vi "Escape.vi"(11 "text":string) -> (3 "escaped text":string)   [LabVIEW 2021, in "HttpServer.lvlib"]
uses:
  HttpServer.lvlib
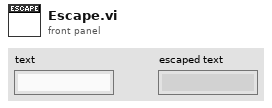
[diagram p1: front panel]
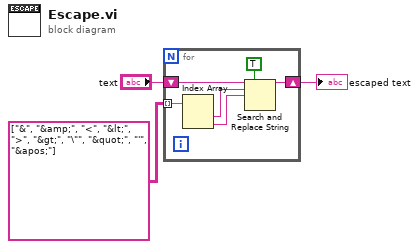
[diagram p0: block diagram]
diagram:
  n1 = for {
    tunnel: string[][] [["&", "&amp;"], ["<", "&lt;"], [">", "&gt;"], ["\"", "&quot;"], ["'", "&apos;"]] -> [w7] mode=indexing
    shift-right: [w4] -> w1
    shift-left: "text" -> [w9]
    n2 = Index Array(array=w7) -> (element #1=w6:string, element #2=w5:string)  [unwired: 2 in]
    n3 = Search and Replace String(replace all?=TRUE ("replace all? (F)"), input string=w9, search string=w6, replace string=w5) -> (result string=w4:string)  [unwired: 4 in, 3 out]
  }
  "escaped text" <- w1
